vi "ReadEnviromentalTemp.vi"() -> (0 "error out":errorcluster, 3 "Probe 1 temperature":dbl format="%.2f")   [LabVIEW 2009]
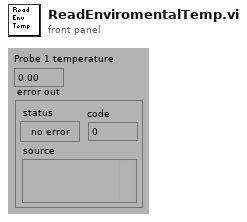
[diagram p1: front panel]
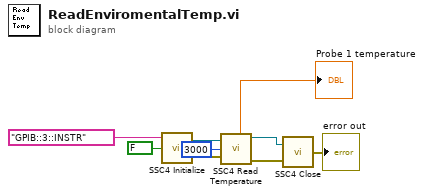
[diagram p0: block diagram]
diagram:
  n1 = call "SSC4 Initialize.vi"("reset"=FALSE, "instrument descriptor"="GPIB::3::INSTR") -> ("error out"=w5:errorcluster, "VISA session"=w6:refnum<visa-resource-name>)  [unwired: 1 in]
  n2 = call "SSC4 Read Temperature.vi"("error in (no error)"=w5, "Command Delay (ms)"=u32 3000, "Visa Session"=w6) -> ("error out"=w2:errorcluster, "Probe 1 temperature"=→"Probe 1 temperature":dbl, "Dup Visa Session"=w3:refnum<visa-resource-name>)  [unwired: 2 in, 1 out]
  n3 = call "SSC4 Close.vi"("error in (no error)"=w2, "VISA session"=w3) -> ("error out"=→"error out":errorcluster)
